vi "Enqueue Message (Array).vi"(6 "Array der Nachrichten hoher Priorität":bool[](array[boolean]), 8 "error in (no error)":T1 caption="Fehler (Eingang, kein Fehler)", 9 "Nachrichtendaten-Array":variant[](array[variant]), 10 "Nachrichten-Array":string[](array[string]), 11 "Nachrichten-Queue":refnum<queue>) -> (0 "error out":T1 caption="Fehler (Ausgang)", 3 "Nachrichten-Queue (Kopie)":refnum<queue>)   [LabVIEW 2014, in "MyQH Message Queue.lvlib"]
doc: "Normale Nachrichten werden an die Queue angehängt. Nachrichten mit hoher Priorität werden an den Anfang der Queue eingefügt."
uses:
  MyQH Message Queue.lvlib
  Message Cluster.ctl
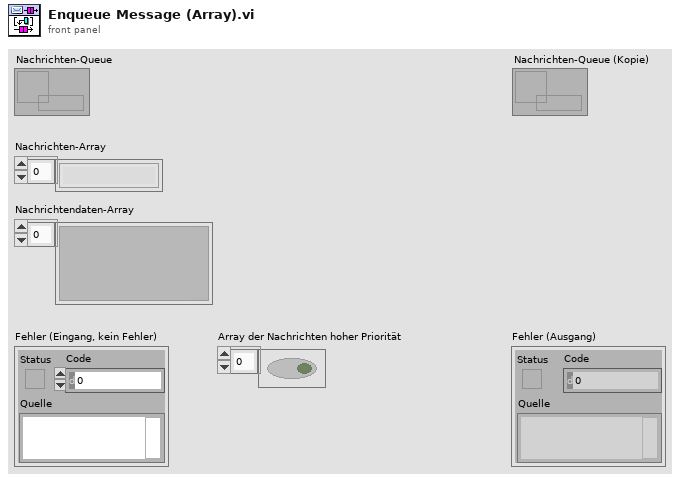
[diagram p1: front panel]
types:
  T1 = cluster{"Status":bool, "Code":i32, "Quelle":string}
  T2 = typedef "MyQH Message Queue.lvlib/Message Cluster.ctl" = cluster{"Nachricht":string, "Nachrichtendaten":variant}
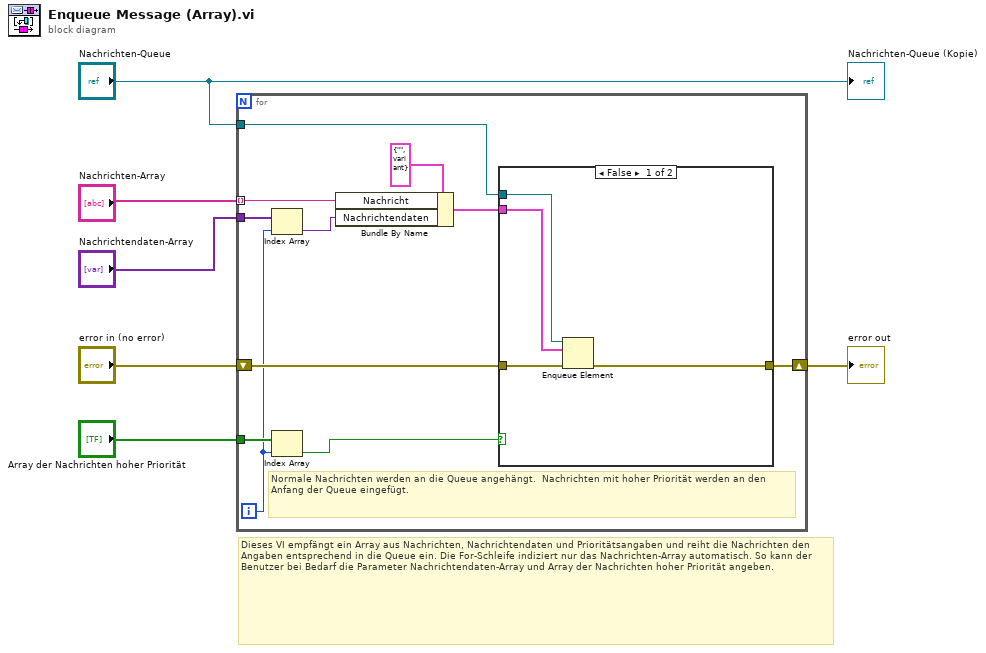
[diagram p0: block diagram]
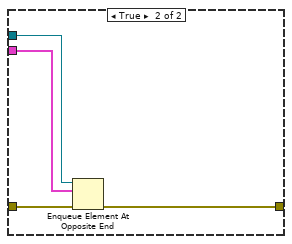
[diagram p2: hidden frame]
diagram:
  # "Dieses VI empfängt ein Array aus Nachrichten, Nachrichtendaten und Prioritätsangaben und reiht die Nachrichten den Angaben entsprechend in die Queue ein. Die For-Schleife indiziert nur das Nachrichten-Array automatisch. So kann der Benutzer bei Bedarf die Parameter Nachrichtendaten-Array und Array der Nachrichten hoher Priorität angeben."
  n1 = for {
    tunnel: "Nachrichten-Array" -> [w16] mode=indexing
    tunnel: "Nachrichtendaten-Array" -> [w11]
    tunnel: "Array der Nachrichten hoher Priorität" -> [w9]
    tunnel: "Nachrichten-Queue" -> [w13]
    shift-right: [w14] -> w2
    shift-left: "error in (no error)" -> [w15]
    i -> [w7]
    # "Normale Nachrichten werden an die Queue angehängt.  Nachrichten mit hoher Priorität werden an den Anfang der Queue eingefügt."
    n2 = Index Array(array=w11, index=w7) -> (element=w10:variant)
    n3 = Index Array(array=w9, index=w7) -> (element=w8:bool)
    n4 = Bundle By Name(cluster=T2 {"Nachricht"="", "Nachrichtendaten"=variant} ("Message Cluster"), "Nachricht"=w16, "Nachrichtendaten"=w10) -> (w12:T2)
    n5 = case shown="False" w8 {
      tunnel: w15 -> [w21 w25]
      tunnel: [w20 w24] -> w14
      tunnel: w13 -> [w19 w23]
      tunnel: w12 -> [w18 w22]
      frame False {
        n6 = Enqueue Element(queue=w19, element=w18, error in (no error)=w21) -> (error out=w20:errorcluster)  [unwired: 1 in, 2 out]
      }
      frame True {
        n7 = Enqueue Element At Opposite End(queue=w23, element=w22, error in (no error)=w25) -> (error out=w24:errorcluster)  [unwired: 1 in, 2 out]
      }
    }
  }
  "error out" <- w2
  "Nachrichten-Queue (Kopie)" <- "Nachrichten-Queue"
